vi "createChannels.vi"(8 "error in (no error)":errorcluster, 11 "DIO64Output in":refnum<class "DIO64Output.lvclass">) -> (0 "error out":errorcluster, 3 "DIO64Output out":refnum<class "DIO64Output.lvclass">)   [LabVIEW 2011, in "Hardware.lvlib" / "Channels.lvlib" / "DIO64Output.lvclass"]
uses:
  DIO64Output.lvclass
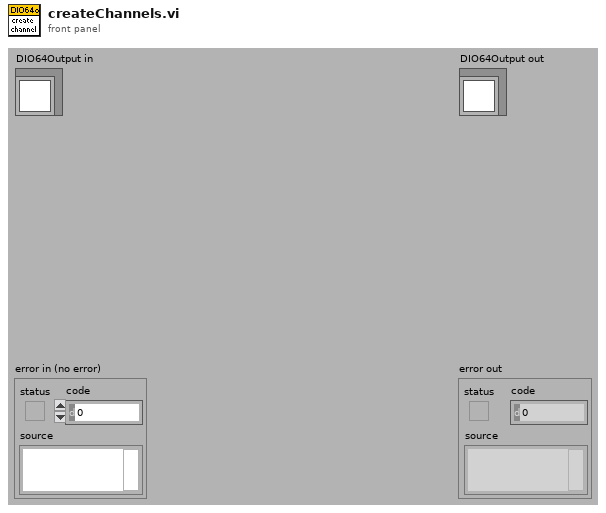
[diagram p1: front panel]
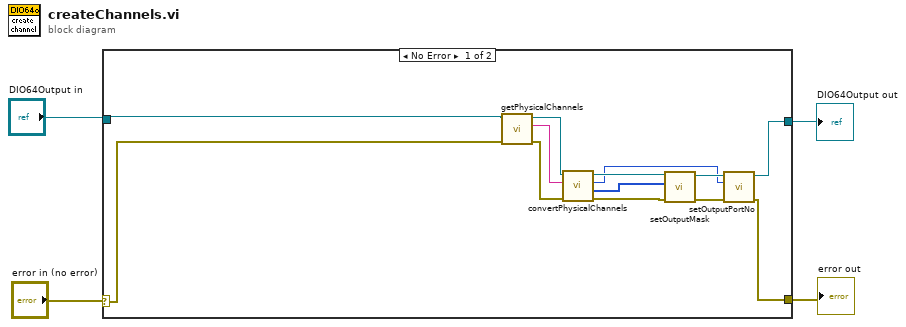
[diagram p0: block diagram]
diagram:
  n1 = case shown="No Error" "error in (no error)" {
    selector: "error in (no error)" -> [w5 w19]
    tunnel: [w14 w19] -> w3
    tunnel: "DIO64Output in" -> [w6 w18]
    tunnel: [w15 w18] -> w1
    frame No Error {
      n2 = call-dynamic "getPhysicalChannels.vi"("error in (no error)"=w5, "DigitalOutput.lvclass in"=w6) -> ("error out"=w11:errorcluster, "Physical Channels"=w12:string, "DigitalOutput.lvclass out"=w13:refnum<class "DIO64Output.lvclass">)  [unwired: 7 in]
      n3 = call "convertPhysicalChannels.vi"("error in (no error)"=w11, "Physical Channels"=w12, "DIO64Output in"=w13) -> ("error out"=w8:errorcluster, "mask"=w9:u16[], "#ports"=w7:u8, "DIO64Output out"=w10:refnum<class "DIO64Output.lvclass">)  [unwired: 5 in]
      n4 = call "setOutputMask.vi"("error in (no error)"=w8, "mask"=w9, "DIO64Output.lvclass in"=w10) -> ("error out"=w16:errorcluster, "DIO64Output.lvclass out"=w17:refnum<class "DIO64Output.lvclass">)  [unwired: 7 in]
      n5 = call "setOutputPortNo.vi"("error in (no error)"=w16, "#ports"=w7, "DIO64Output.lvclass in"=w17) -> ("error out"=w14:errorcluster, "DIO64Output.lvclass out"=w15:refnum<class "DIO64Output.lvclass">)  [unwired: 7 in]
    }
    frame Error {
    }
  }
  "error out" <- w3
  "DIO64Output out" <- w1
